vi "Host.vi"() -> ()   [LabVIEW 2017]
uses:
  <vilib>/NI/STM/TCP/TCP Read Options.ctl
  TypeDefs/Data for Logging.ctl
  TypeDefs/ClientStatusData.ctl
  <vilib>/NI/STM/TCP/Read Meta Data (TCP Ref).vi
  <vilib>/NI/STM/TCP/Get Connection Reference (TCP).vi
  <vilib>/NI/STM/TCP/Read Meta Data (TCP Clst).vi
  <vilib>/NI/STM/TCP/Write Message (TCP).vi
  <vilib>/NI/STM/TCP/Read Message (TCP).vi
  <vilib>/NI/STM/NI STM.lvlib
panel:
  out "RECENT PLAYERS":string[](array[string])
  out "X POSITION":cluster{dbl, dbl}(graph)
  out "Y POSITION":cluster{dbl, dbl}(graph)
  out "DAVE":cluster{dbl[], dbl[]}[](graph)
  in  "assistance":bool
  out "error  out":errorcluster
  in  "stop":bool
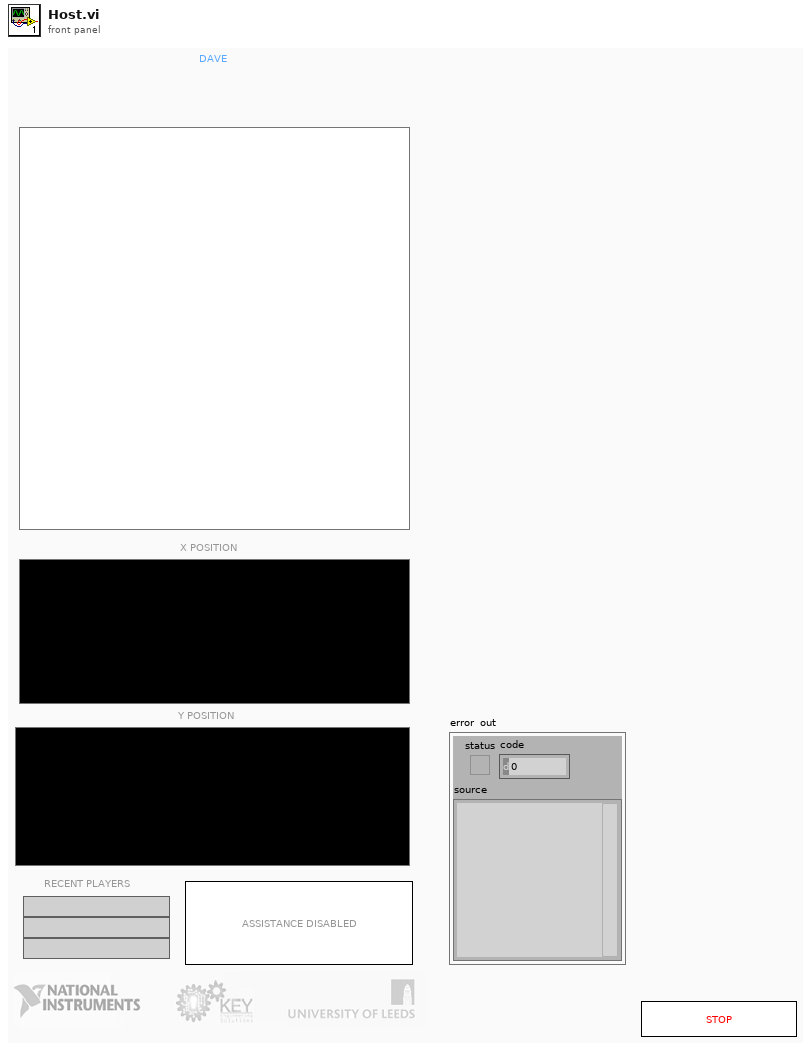
[diagram p1: front panel]
types:
  T1 = enum16{"open", "replace", "create", "open or create", "replace or create", "replace or create with confirmation"}
  T2 = typedef "NI STM.lvlib/TCP Connection Info.ctl" = cluster{"connection ID":refnum<k5>, "meta data":T3[]}
  T3 = typedef "NI STM.lvlib/MetaDataElement.ctl" = string
  T4 = typedef "NI STM.lvlib/TCP Read Options.ctl" = cluster{"ignore timeout error":bool, "timeout ms (1000)":i32}
  T5 = typedef "Data for Logging.ctl" = cluster{"end effector x (mm)":dbl, "end effector y (mm)":dbl, "target x (mm)":dbl, "target y (mm)":dbl, "Theta 1":dbl, "Theta 2":dbl, "Omega 1":dbl, "Omega 2":dbl, "Timestamp":dbl}
  T6 = typedef "ClientStatusData.ctl" = cluster{"gameState":u16, "playerName":string, "playerScore":dbl, "gameUnits":string}
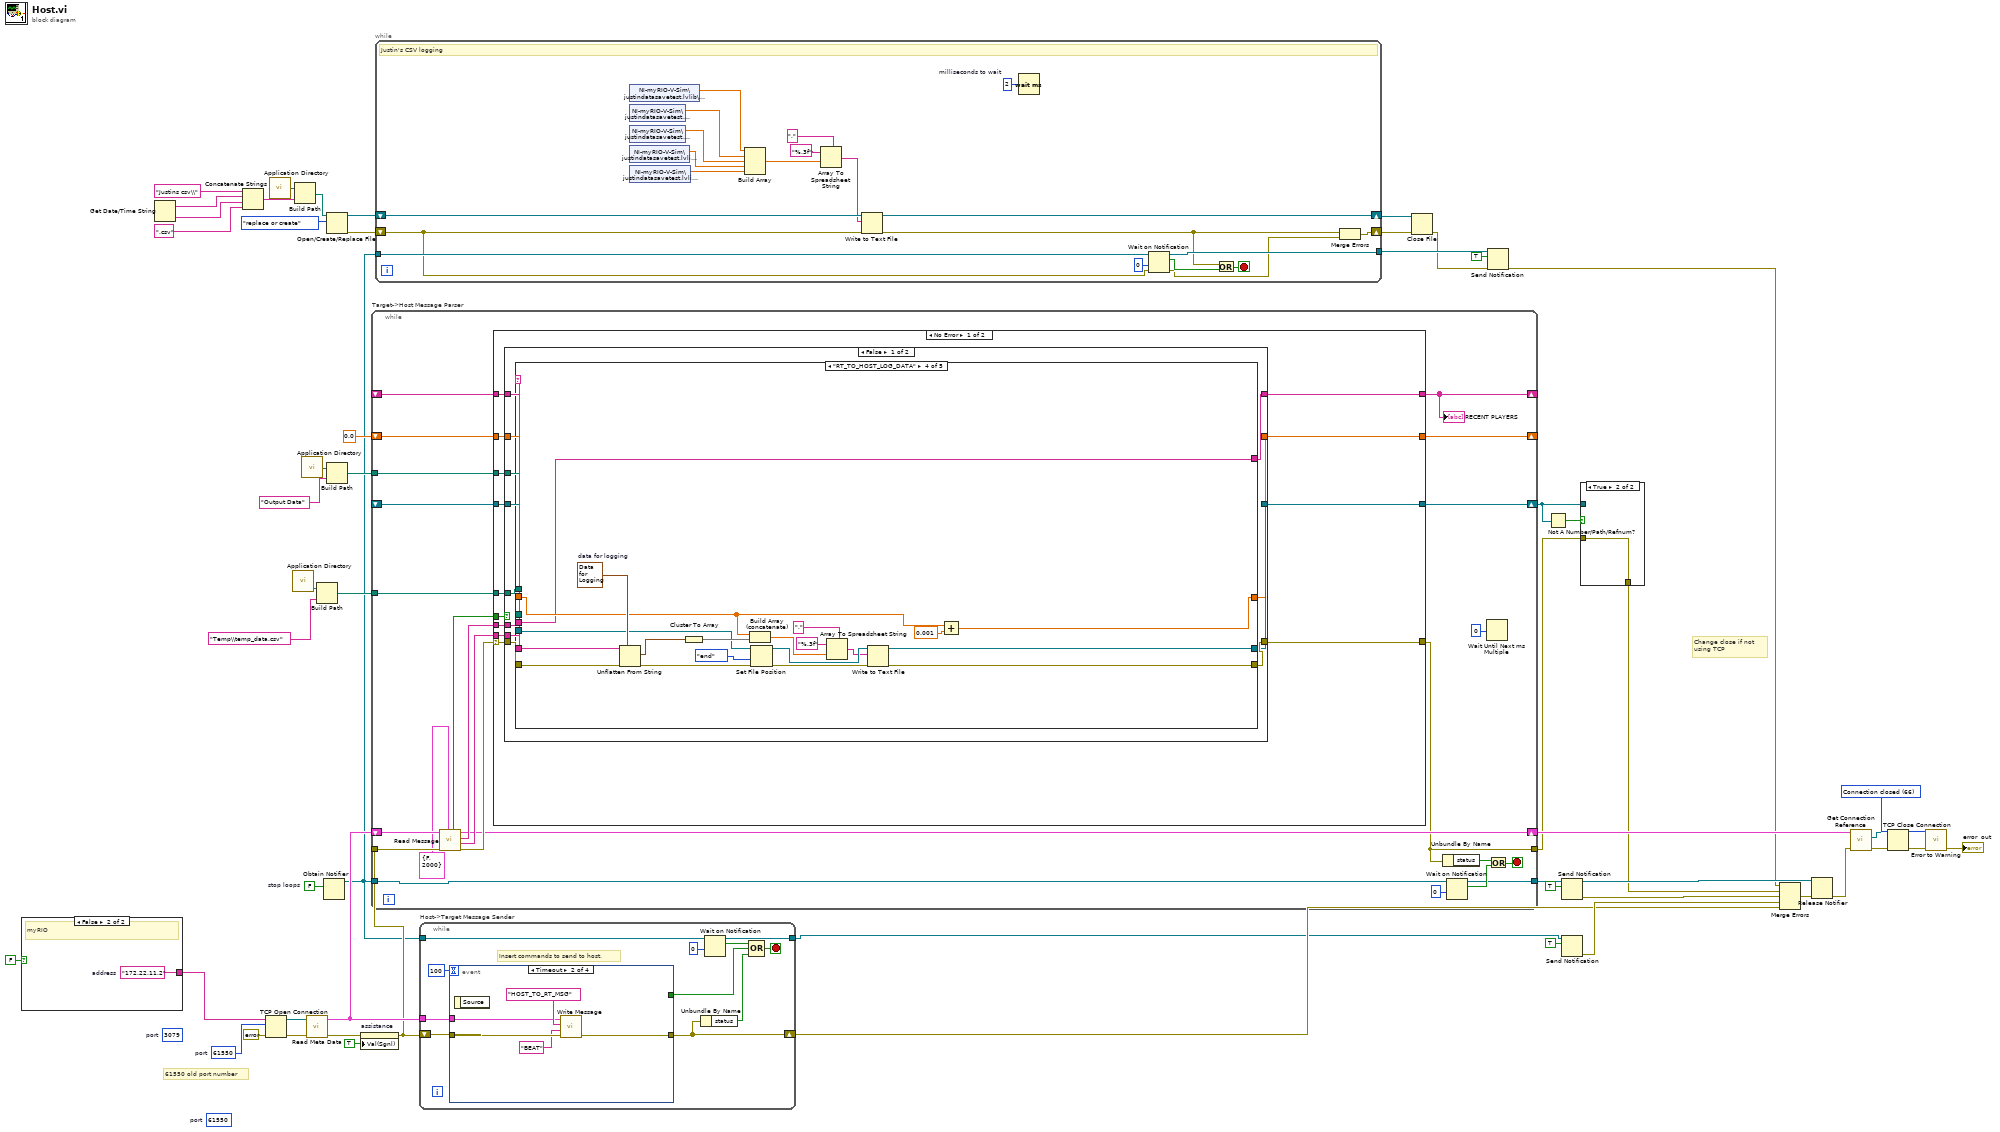
[diagram p0: block diagram]
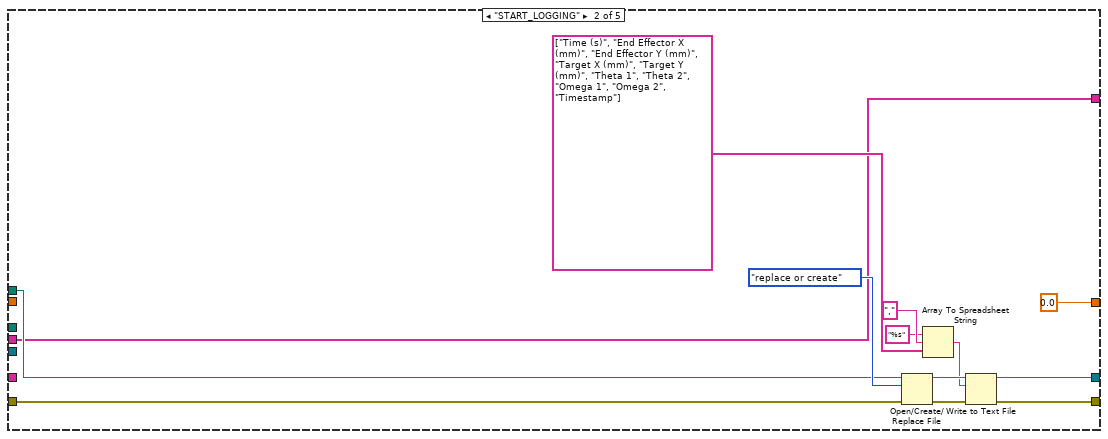
[diagram p3: hidden frame]
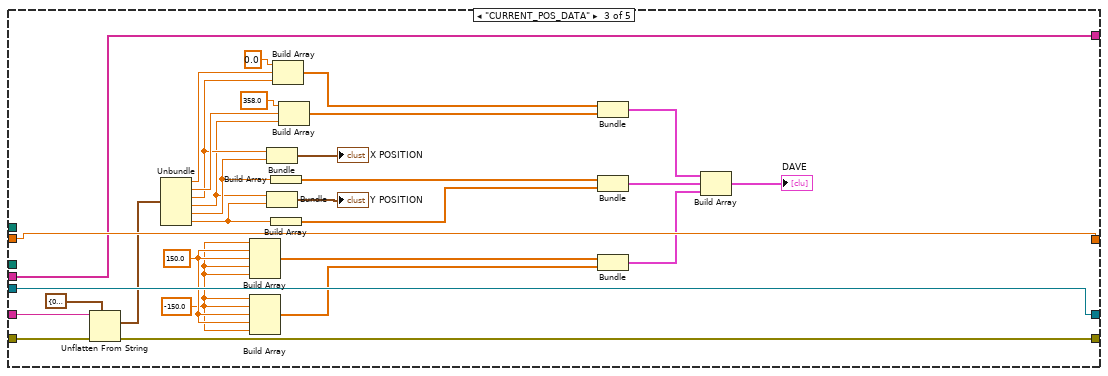
[diagram p4: hidden frame]
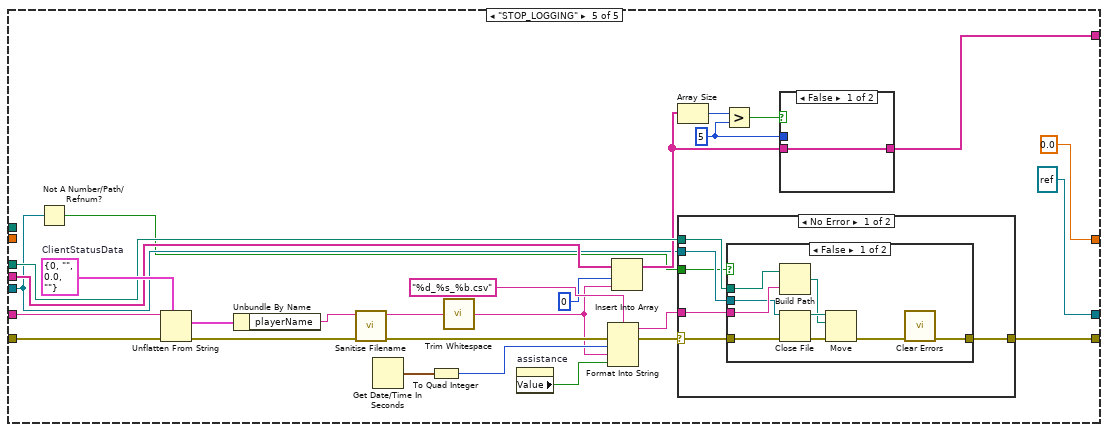
[diagram p5: hidden frame]
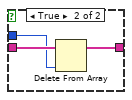
[diagram p8: hidden frame]
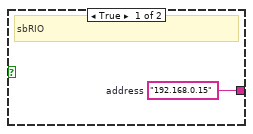
[diagram p11: hidden frame]
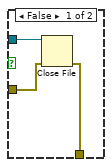
[diagram p12: hidden frame]
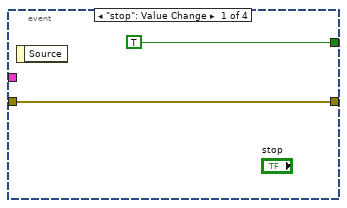
[diagram p13: hidden frame]
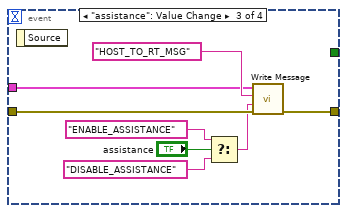
[diagram p14: hidden frame]
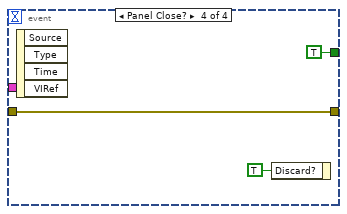
[diagram p15: hidden frame]
diagram:
  (unwired) u16 61550  # port
  w19 = u16 61550  # port
  w40 = FALSE  # stop loops
  w51 = 66 items=["No Error", "Argument Error", "Memory Full", "Out of Zone", "End of File", "File Already Open", "Generic File IO Error", "File Not Found", "File Permission Error", "Disk Full", "Duplicate Path", "Too Many Files Open", "Not Enabled", "Resource File Not Found", "Cannot Add Resource", "Resource Not Found", "Image Not Found", "Image Memory Error", "Pen Does Not Exist", "Config Bad Type", "Config Token Not Found", "Config Parse Error", "Config Memory Error", "Bad External Code Format", "Bad External Code Offset", "External Code Not Present", "Null Window", "Destroy Window Mixup", "Null Menu", "Print Aborted", "Bad Print Record", "Print Driver Error", "Windows Error During Print", "Memory Error During Print", "Print Dialog Error", "Generic Print Error", "Invalid Device Refnum", "Device Not Found", "Device Parameter Error", "Device Unit Error", "Can't Open Device", "Device Call Aborted", "Generic Error", "Cancelled By User", "Object ID Too Low", "Object ID Too High", "Object Not In Heap", "Unknown Heap", "Bad DefProc ID", "DefProc Not In Table", "Message Out Of Range", "Null Method", "Unknown Message", "Manager Call Not Supported", "Bad address", "Connection In progress", "Connection timed out", "Connection is already in progress", "Network attribute not supported", "Network error", "Address in use", "System out of memory", "Connection aborted", "Connection refused", "Connection is not connected", "Connection is already connected", "Connection closed", "Initialize error (interapplication manager)", "Bad occurrence", "Wait on unbound occurrence handler", "Occurrence queue overflow", "Bad path", "Semaphore not signaled", "Unrecognized type (interapplication manager)"] ("1st Error to Convert")
  (unwired) u16 3079  # port
  # "61550 old port number"
  # "Change close if not using TCP"
  n1 = case shown="False" FALSE {
    tunnel: [w56 w57] -> w55
    frame True {
      w56 = "192.168.0.15"  # address
      # "sbRIO"
    }
    frame False {
      w57 = "172.22.11.2"  # address
      # "myRIO"
    }
  }
  n2 = Get Date/Time String() -> (date string=w5:string, time string=w4:string)  [unwired: 3 in]
  n3 = Concatenate Strings("Justins csv\\" ("name or relative path"), w5, w4, ".csv" ("string")) -> (w2:string)
  n4 = TCP Open Connection(address=w55, remote port or service name=w19, error in (no error)=errorcluster {"status"=FALSE, "code"=0, "source"=""}) -> (connection ID=w35:refnum<k5>, error out=w34:errorcluster)  [unwired: 2 in]
  n5 = call <vilib>:"Application Directory.vi"() -> ("Application Directory"=w7:path)
  n6 = call <vilib>:"Application Directory.vi"() -> ("Application Directory"=w32:path)
  n7 = Build Path(base path=w7, name or relative path=w2) -> (appended path=w1:path)
  n8 = call <vilib>:"Application Directory.vi"() -> ("Application Directory"=w30:path)
  n9 = call-poly <vilib>:"Read Meta Data.vi"("error in"=w34, "connection ID"=w35) -> ("error out"=w25:errorcluster, "connection info out"=w38:T2)  [unwired: 1 in, 7 out]
  n10 = Build Path(base path=w32, name or relative path="Temp\\temp_data.csv") -> (appended path=w31:path)
  n11 = Obtain Notifier(notification data type=w40) -> (notifier out=w14:refnum<notifier>)  [unwired: 3 in, 2 out]
  n12 = Open/Create/Replace File(file path (use dialog)=w1, operation (0:open)=T1."replace or create") -> (refnum out=w16:refnum<file>, error out=w15:errorcluster)  [unwired: 4 in, 1 out]
  n13 = Build Path(base path=w30, name or relative path="Output Data") -> (appended path=w28:path)
  n14 = property on="assistance" class="Bool (strict)"(error in=w25, "Val(Sgnl)"=TRUE ("Value (Signaling)")) -> (error out=w24:errorcluster)  [unwired: 1 in, 1 out]
  n15 = while "Target->Host Message Parser" {
    tunnel: w14 -> [w74]
    tunnel: [w70] -> w41
    shift-right: [w75] -> w39
    shift-left: w38 -> [w81]
    tunnel: w31 -> [w66]
    tunnel: w28 -> [w65]
    shift-right: [w64] -> w22
    shift-left: _ -> [w63]
    shift-right: [w61] -> _
    shift-left: 0.0 -> [w62]
    shift-right: [w59] -> _
    shift-left: _ -> [w60]
    tunnel: w24 -> [w80]
    tunnel: [w68] -> w18
    stop <- w71 stop-if-true
    n16 = call-poly <vilib>:"Read Message.vi"("options"=T4 {"ignore timeout error"=FALSE, "timeout ms (1000)"=2000}, "error in"=w80, "connection info in"=w81) -> ("error out"=w76:errorcluster, "name"=w79:T3, "data string"=w78:string, "connection info out"=w75:T2, "timed out?"=w77:bool)  [unwired: 2 in, 2 out]
    n17 = case shown="No Error" w76 {
      selector: w76 -> [w91 w230]
      tunnel: w79 -> [w94 _]
      tunnel: w78 -> [w93 _]
      tunnel: w77 -> [w92 _]
      tunnel: [w90 w230] -> w68
      tunnel: w66 -> [w89 _]
      tunnel: w65 -> [w88 _]
      tunnel: [w87 w229] -> w64
      tunnel: w63 -> [w86 w229]
      tunnel: w62 -> [w85 w228]
      tunnel: [w84 w228] -> w61
      tunnel: w60 -> [w83 w227]
      tunnel: [w82 w227] -> w59
      frame No Error {
        n18 = case shown="False" w92 {
          tunnel: w94 -> [w103 _]
          tunnel: w93 -> [w106 _]
          tunnel: w91 -> [w105 w226]
          tunnel: [w104 w226] -> w90
          tunnel: w89 -> [w102 _]
          tunnel: w88 -> [w101 _]
          tunnel: [w100 w225] -> w87
          tunnel: w86 -> [w99 w225]
          tunnel: w85 -> [w98 w224]
          tunnel: [w97 w224] -> w84
          tunnel: w83 -> [w96 w223]
          tunnel: [w95 w223] -> w82
          frame False {
            n19 = case shown="\"RT_TO_HOST_LOG_DATA\"" w103 {
              tunnel: w106 -> [_ _ w150 w171 w199]
              tunnel: w105 -> [w108 w122 w149 w173 w201]
              tunnel: [w108 w119 w148 w157 w175] -> w104
              tunnel: w102 -> [_ w121 _ _ _]
              tunnel: w101 -> [_ _ _ _ w193]
              tunnel: [w110 w118 w152 w156 refnum<file> refnum ("refnum out")] -> w100
              tunnel: w99 -> [w110 _ w152 w155 w177]
              tunnel: w98 -> [w109 _ w153 w166 _]
              tunnel: [w109 0.0 w153 w168 0.0] -> w97
              tunnel: w96 -> [w107 w111 w127 w154 w185]
              tunnel: [w107 w111 w127 w154 w180] -> w95
              frame Default {
              }
              frame "START_LOGGING" {
                n20 = Open/Create/Replace File(file path (use dialog)=w121, error in=w122, operation (0:open)=T1."replace or create") -> (refnum out=w114:refnum<file>, error out=w115:errorcluster)  [unwired: 3 in, 1 out]
                n21 = Array To Spreadsheet String(delimiter (Tab)=",", array=string[] ["Time (s)", "End Effector X (mm)", "End Effector Y (mm)", "Target X (mm)", "Target Y (mm)", "Theta 1", "Theta 2", "Omega 1", "Omega 2", "Timestamp"], 3:"%s" ("format string")) -> (spreadsheet string=w113:string)
                n22 = Write to Text File(file (use dialog)=w114, text=w113, error in=w115) -> (refnum out=w118:refnum<file>, error out=w119:errorcluster)  [unwired: 1 in, 1 out]
              }
              frame "CURRENT_POS_DATA" {
                w132 = -150.0
                w133 = 150.0
                n23 = Unflatten From String(type=cluster{dbl, dbl, dbl, dbl, dbl, dbl} {0.0, 0.0, 0.0, 0.0, 0.0, 0.0}, binary string=w150, error in (no error)=w149) -> (value=w147:cluster{dbl, dbl, dbl, dbl, dbl, dbl}, error out=w148:errorcluster)  [unwired: 2 in, 1 out]
                n24 = Unbundle(w147) -> (w144:dbl, w143:dbl, w125:dbl, w124:dbl, w130:dbl, w131:dbl)
                n25 = Build Array(w132, w133, w133, w132, w132) -> (w135:dbl[])
                n26 = Build Array(w132, w132, w133, w133, w132) -> (w134:dbl[])
                n27 = Bundle(w125, w130) -> (→"X POSITION":cluster{dbl, dbl})  [unwired: 1 in]
                n28 = Bundle(w124, w131) -> (→"Y POSITION":cluster{dbl, dbl})  [unwired: 1 in]
                n29 = Build Array(w130) -> (w138:dbl[])
                n30 = Build Array(w131) -> (w137:dbl[])
                n31 = Build Array(0.0 ("element"), w144, w125) -> (w142:dbl[])
                n32 = Build Array(358.0 ("element"), w143, w124) -> (w141:dbl[])
                n33 = Bundle(w142, w141) -> (w140:cluster{dbl[], dbl[]})  [unwired: 1 in]
                n34 = Bundle(w138, w137) -> (w136:cluster{dbl[], dbl[]})  [unwired: 1 in]
                n35 = Bundle(w135, w134) -> (w126:cluster{dbl[], dbl[]})  [unwired: 1 in]
                n36 = Build Array(w140, w136, w126) -> (→"DAVE":cluster{dbl[], dbl[]}[])
              }
              frame "RT_TO_HOST_LOG_DATA" {
                w172 = T5 {"end effector x (mm)"=0.0, "end effector y (mm)"=0.0, "target x (mm)"=0.0, "target y (mm)"=0.0, "Theta 1"=0.0, "Theta 2"=0.0, "Omega 1"=0.0, "Omega 2"=0.0, "Timestamp"=0.0}  # data for logging
                n37 = Unflatten From String(type=w172, binary string=w171, error in (no error)=w173) -> (value=w170:T5, error out=w162:errorcluster)  [unwired: 2 in, 1 out]
                n38 = Cluster To Array(cluster=w170) -> (array=w167:dbl[])
                n39 = Build Array (concatenate)(w166, w167) -> (w165:dbl[])
                n40 = Set File Position(refnum=w155, from (0:start)=enum16{"start", "end", "current"}."end", error in=w162) -> (refnum out=w159:refnum<file>, error out=w160:errorcluster)  [unwired: 1 in]
                n41 = Array To Spreadsheet String(delimiter (Tab)=",", array=w165, 3:"%.3f" ("format string")) -> (spreadsheet string=w158:string)
                n42 = Write to Text File(file (use dialog)=w159, text=w158, error in=w160) -> (refnum out=w156:refnum<file>, error out=w157:errorcluster)  [unwired: 1 in, 1 out]
                n43 = Add(x=w166, y=0.001) -> (x+y=w168:dbl)
              }
              frame "STOP_LOGGING" {
                w181 = 5 ("y")
                w200 = T6 {"gameState"=0, "playerName"="", "playerScore"=0.0, "gameUnits"=""}  # ClientStatusData
                n44 = Not A Number/Path/Refnum?(number/path/refnum=w177) -> (NaN/Path/Refnum?=w176:bool)
                n45 = Unflatten From String(type=w200, binary string=w199, error in (no error)=w201) -> (value=w197:T6, error out=w189:errorcluster)  [unwired: 2 in, 1 out]
                n46 = Unbundle By Name(w197) -> ("playerName"=w187:string)
                n47 = call "Sanitise Filename.vi"("error in"=w189, "input filename"=w187) -> ("error out"=w188:errorcluster, "output filename"=w186:string)  [unwired: 8 in]
                n48 = Get Date/Time In Seconds() -> (seconds since 1Jan1904=w196:timestamp)
                n49 = To Quad Integer(1:w196) -> (0:w195:i64)
                n50 = call <vilib>:"Trim Whitespace.vi"("string"=w186) -> ("trimmed string"=w179:string)  [unwired: 1 in]
                n51 = property on="assistance" class="Bool (strict)"() -> ("Value"=w174:bool)  [unwired: 2 in, 2 out]
                n52 = Format Into String(format string="%d_%s_%b.csv", error in=w188, w195, w179, w174) -> (resulting string=w192:string, error out=w190:errorcluster)  [unwired: 1 in]
                n53 = Insert Into Array(array=w185, index=0, new element=w179) -> (w182:string[])
                n54 = Array Size(array=w182) -> (size(s)=w184:i32)
                n55 = case shown="No Error" w190 {
                  selector: w190 -> [w205 w218]
                  tunnel: w193 -> [w207 _]
                  tunnel: w192 -> [w206 _]
                  tunnel: w177 -> [w204 _]
                  tunnel: w176 -> [w203 _]
                  tunnel: [w202 w218] -> w175
                  frame No Error {
                    n56 = case shown="False" w203 {
                      tunnel: w207 -> [w216 _]
                      tunnel: w206 -> [w215 _]
                      tunnel: w205 -> [w212 w217]
                      tunnel: w204 -> [w210 _]
                      tunnel: [w208 w217] -> w202
                      frame False {
                        n57 = Build Path(base path=w216, name or relative path=w215) -> (appended path=w213:path)
                        n58 = Close File(refnum=w210, error in=w212) -> (path=w214:path, error out=w211:errorcluster)
                        n59 = Move(source path=w214, error in=w211, 10:w213) -> (error out=w209:errorcluster)  [unwired: 2 in, 2 out]
                        n60 = call <vilib>:"Clear Errors.vi"("error in (no error)"=w209) -> ("error out"=w208:errorcluster)  [unwired: 5 in, 1 out]
                      }
                      frame True {
                      }
                    }
                  }
                  frame Error {
                  }
                }
                n61 = Greater?(x=w184, y=w181) -> (0:w183:bool)
                n62 = case shown="False" w183 {
                  tunnel: w182 -> [w219 w222]
                  tunnel: w181 -> [_ w221]
                  tunnel: [w219 w220] -> w180
                  frame False {
                  }
                  frame True {
                    n63 = Delete From Array(array=w222, index=w221) -> (array with subset deleted=w220:string[])  [unwired: 1 in, 1 out]
                  }
                }
              }
            }
          }
          frame True {
          }
        }
      }
      frame Error {
      }
    }
    "RECENT PLAYERS" <- w59
    n64 = Unbundle By Name(w68) -> ("status"=w69:bool)
    n65 = Wait on Notification(notifier=w74, timeout in ms (-1)=0) -> (notifier out=w70:refnum<notifier>, notification=w72:bool)  [unwired: 2 in, 2 out]
    n66 = Wait Until Next ms Multiple(millisecond multiple=u32 0) -> ()  [unwired: 1 out]
    n67 = Or(x=w69, y=w72) -> (x .or. y?=w71:bool)
  }
  n68 = while {
    shift-right: [w241] -> w10
    shift-left: w16 -> [w250]
    shift-right: [w243] -> w9
    shift-left: w15 -> [w245]
    tunnel: w14 -> [w247]
    tunnel: [w246] -> w12
    stop <- w251 stop-if-true
    w231 = u32 2  # milliseconds to wait
    # "Justin's CSV logging"
    n69 = shared-variable "NI-myRIO-V-Sim\\justindatasavetest.lvlib\\timestamp"() -> (w240:dbl)  [unwired: 1 in, 1 out]
    n70 = shared-variable "NI-myRIO-V-Sim\\justindatasavetest.lvlib\\targetx"() -> (w239:dbl)  [unwired: 1 in, 1 out]
    n71 = shared-variable "NI-myRIO-V-Sim\\justindatasavetest.lvlib\\targety"() -> (w238:dbl)  [unwired: 1 in, 1 out]
    n72 = shared-variable "NI-myRIO-V-Sim\\justindatasavetest.lvlib\\currentx"() -> (w237:dbl)  [unwired: 1 in, 1 out]
    n73 = shared-variable "NI-myRIO-V-Sim\\justindatasavetest.lvlib\\currenty"() -> (w236:dbl)  [unwired: 1 in, 1 out]
    n74 = Build Array(w240, w239, w238, w237, w236) -> (w233:dbl[])
    n75 = Array To Spreadsheet String(delimiter (Tab)=",", array=w233, 3:"%.3f" ("format string")) -> (spreadsheet string=w232:string)
    n76 = Write to Text File(file (use dialog)=w250, text=w232, error in=w245) -> (refnum out=w241:refnum<file>, error out=w244:errorcluster)  [unwired: 1 in, 1 out]
    n77 = Wait (ms)(milliseconds to wait=w231) -> ()  [unwired: 1 out]
    n78 = Wait on Notification(notifier=w247, timeout in ms (-1)=0, error in (no error)=w245) -> (notifier out=w246:refnum<notifier>, notification=w248:bool, error out=w242:errorcluster)  [unwired: 1 in, 1 out]
    n79 = Or(x=w244, y=w248) -> (x .or. y?=w251:bool)
    n80 = Merge Errors(w244, w242) -> (w243:errorcluster)
  }
  n81 = while "Host->Target Message Sender" {
    shift-right: [w254] -> w45
    shift-left: w24 -> [w262]
    tunnel: w38 -> [w261]
    tunnel: w14 -> [w258]
    tunnel: [w255] -> w43
    stop <- w256 stop-if-true
    # "Insert commands to send to host."
    n82 = event shown="[1] Timeout" {
      selector: _ -> [_ _ _ _]
      dyn-events: _ -> [_ _ _ _]
      timeout: 100 -> [_ _ _ _]
      tunnel: w261 -> [_ w266 w274 _]
      tunnel: w262 -> [w264 w269 w277 w278]
      tunnel: [TRUE ("stop") _ _ TRUE ("stop")] -> w253
      tunnel: [w264 w268 w276 w278] -> w254
      event "stop": Value Change {
        n83 = event-data() -> ()  [unwired: 2 out]
      }
      event Timeout {
        n84 = event-data() -> ()  [unwired: 2 out]
        n85 = call-poly <vilib>:"Write Message.vi"("error in"=w269, "data"="BEAT", "name"="HOST_TO_RT_MSG", "connection info in"=w266) -> ("error out"=w268:errorcluster)  [unwired: 1 in, 6 out]
      }
      event "assistance": Value Change {
        n86 = event-data() -> ()  [unwired: 2 out]
        n87 = Select(t="ENABLE_ASSISTANCE" ("data"), s="assistance", f="DISABLE_ASSISTANCE" ("data")) -> (s? t:f=w270:string)
        n88 = call-poly <vilib>:"Write Message.vi"("error in"=w277, "data"=w270, "name"="HOST_TO_RT_MSG", "connection info in"=w274) -> ("error out"=w276:errorcluster)  [unwired: 1 in, 6 out]
      }
      event Panel Close? {
        n89 = event-data() -> ()  [unwired: 5 out]
        n90 = event-data("Discard?"=TRUE) -> ()  [unwired: 1 in, 1 out]
      }
    }
    n91 = Unbundle By Name(w254) -> ("status"=w252:bool)
    n92 = Wait on Notification(notifier=w258, timeout in ms (-1)=0) -> (notifier out=w255:refnum<notifier>, notification=w260:bool)  [unwired: 2 in, 2 out]
    n93 = Compound Arithmetic op=OR(w260, w253, w252) -> (w256:bool)
  }
  n94 = Close File(refnum=w10, error in=w9) -> (error out=w8:errorcluster)  [unwired: 1 out]
  n95 = Send Notification(notification=TRUE, notifier=w12, error in (no error)=w8) -> (error out=w11:errorcluster)  [unwired: 1 out]
  n96 = Not A Number/Path/Refnum?(number/path/refnum=w22) -> (NaN/Path/Refnum?=w23:bool)
  n97 = Send Notification(notification=TRUE, notifier=w41) -> (notifier out=w48:refnum<notifier>, error out=w47:errorcluster)  [unwired: 1 in]
  n98 = Send Notification(notification=TRUE, notifier=w43) -> (error out=w46:errorcluster)  [unwired: 1 in, 1 out]
  n99 = case shown="True" w23 {
    tunnel: w22 -> [w283 _]
    tunnel: w18 -> [w282 w284]
    tunnel: [w281 w284] -> w21
    frame False {
      n100 = Close File(refnum=w283, error in=w282) -> (error out=w281:errorcluster)  [unwired: 1 out]
    }
    frame True {
    }
  }
  n101 = Merge Errors(w11, w21, w47, w46, w45) -> (w49:errorcluster)
  n102 = Release Notifier(notifier=w48, error in (no error)=w49) -> (error out=w50:errorcluster)  [unwired: 1 in, 2 out]
  n103 = call-poly <vilib>:"Get Connection Reference.vi"("error in"=w50, "connection info in"=w39) -> ("error out"=w37:errorcluster, "connection ID out"=w36:refnum<k5>)  [unwired: 8 out]
  n104 = TCP Close Connection(connection ID=w36, error in (no error)=w37) -> (error out=w52:errorcluster)  [unwired: 2 out]
  n105 = call <vilib>:"Error to Warning.vi"("1st Error to Convert"=w51, "error in"=w52) -> ("warning out"=→"error  out":errorcluster)  [unwired: 3 in, 10 out]
